vi "Get_Total_Amount.vi"(0 "Vending_data":T1, 5 "Inserted_Cash?":bool=TRUE) -> (4 "Total_Amount":i32, 6 "Is_Amount_Enough?":bool)   [LabVIEW 2023]
doc: "Used to get the total amount in the bundle."
uses:
  Controls/Vending_Data.ctl
  Controls/INI_Data.ctl
  Controls/Total_Cash_Count.ctl
  Controls/Inserted_Cash_Count.ctl
  Controls/Controls_Referece.ctl
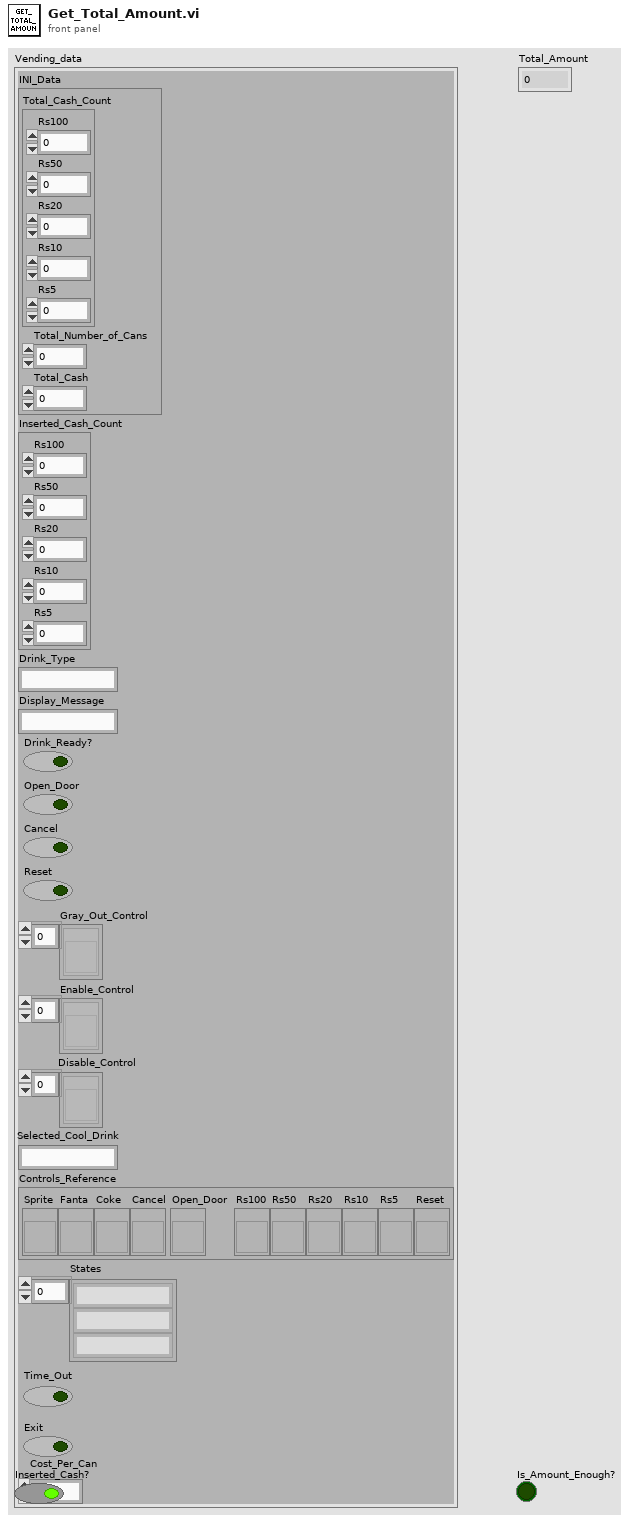
[diagram p1: front panel]
types:
  T1 = typedef "Vending_Data.ctl" = cluster{"INI_Data":T2, "Inserted_Cash_Count":T4, "Drink_Type":string, "Display_Message":string, "Drink_Ready?":bool, "Open_Door":bool, "Cancel":bool, "Reset":bool, "Gray_Out_Control":refnum<vi>[], "Enable_Control":refnum<vi>[], "Disable_Control":refnum<vi>[], "Selected_Cool_Drink":string, "Controls_Reference":T5, "States":string[], "Time_Out":bool, "Exit":bool, "Cost_Per_Can":i32}
  T2 = typedef "INI_Data.ctl" = cluster{"Total_Cash_Count":T3, "Total_Number_of_Cans":i32, "Total_Cash":i32}
  T3 = typedef "Total_Cash_Count.ctl" = cluster{"Rs100":i32, "Rs50":i32, "Rs20":i32, "Rs10":i32, "Rs5":i32}
  T4 = typedef "Inserted_Cash_Count.ctl" = cluster{"Rs100":i32, "Rs50":i32, "Rs20":i32, "Rs10":i32, "Rs5":i32}
  T5 = typedef "Controls_Referece.ctl" = cluster{"Sprite":refnum<vi>, "Fanta":refnum<vi>, "Coke":refnum<vi>, "Cancel":refnum<vi>, "Open_Door":refnum<vi>, "Rs100":refnum<vi>, "Rs50":refnum<vi>, "Rs20":refnum<vi>, "Rs10":refnum<vi>, "Rs5":refnum<vi>, "Reset":refnum<vi>}
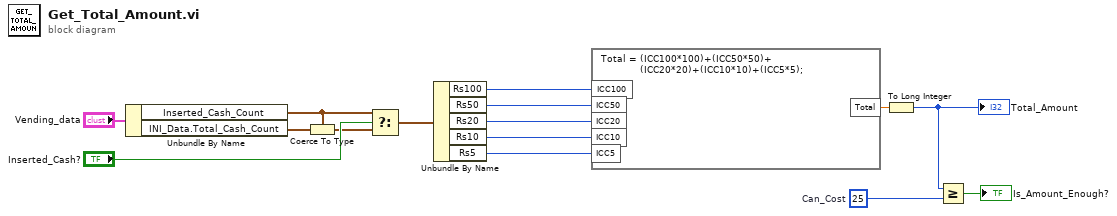
[diagram p0: block diagram]
diagram:
  w15 = 25  # Can_Cost
  n1 = Unbundle By Name("Vending_data") -> ("Inserted_Cash_Count"=w1:T4, "INI_Data.Total_Cash_Count"=w5:T3)
  n2 = Coerce To Type(0:w5, 1:w1) -> (2:w2:T4)
  n3 = Select(t=w1, s="Inserted_Cash?", f=w2) -> (s? t:f=w4:T4)
  n4 = Unbundle By Name(w4) -> ("Rs100"=w9:i32, "Rs50"=w10:i32, "Rs20"=w11:i32, "Rs10"=w12:i32, "Rs5"=w13:i32)
  n5 = formula code="Total = (ICC100*100)+(ICC50*50)+\n             (ICC20*20)+(ICC10*10)+(ICC5*5);"("ICC100"=w9, "ICC50"=w10, "ICC20"=w11, "ICC10"=w12, "ICC5"=w13) -> ("Total"=w14:dbl)
  n6 = To Long Integer(number=w14) -> (32bit integer=w7:i32)
  "Total_Amount" <- w7
  n7 = Greater Or Equal?(x=w7, y=w15) -> (x >= y?=→"Is_Amount_Enough?":bool)
